vi "Robot Global Data.vi"() -> ()   [LabVIEW 2017]
doc: "This global VI can contain as many global variables as you need. Place a control on the panel, give it a good name. To read or write to it from a VI, drag the icon to the diagram of that VI. You can also drag from the project. Click on the node to change which global you access. You shouldn't have multiple locations writing to a global or it will cause a race-condition."
uses:
  <vilib>/Rock Robotics/WPI/Camera/WPI_CameraImageSize.ctl
  <vilib>/Rock Robotics/WPI/DriverStation/WPI_DriverStationRobotMode2.ctl
panel:
  in  "SweetSpot":dbl=0.4
  out "WristSet":dbl
  out "LiftSet":dbl
  out "TempWrist":dbl
  out "WristVelocity":dbl
  out "WristDistance":dbl
  in  "WristDistanceArr":dbl[](array[numeric])
  in  "WristVelocityArr":dbl[](array[numeric])
  out "LiftVelocity":dbl
  out "LiftDistance":dbl
  in  "LiftDistanceArr":dbl[](array[numeric])
  in  "LiftVelocityArr":dbl[](array[numeric])
  in  "Cube Found?":bool
  in  "LiftSet?":bool
  out "AvgVel":dbl
  out "AvgDist":dbl
  out "YawVelocity":dbl
  out "Yaw":dbl
  in  "NavXArr":dbl[](array[numeric])
  out "RightVelocity":dbl
  out "RightDistance":dbl
  out "LeftVelocity":dbl
  out "LeftDistance":dbl
  in  "RightDistanceArr":dbl[](array[numeric])
  in  "LeftDistanceArr":dbl[](array[numeric])
  in  "RightVelocityArr":dbl[](array[numeric])
  in  "LeftVelocityArr":dbl[](array[numeric])
  out "IntakeTime":dbl
  out "IntakeSwitch":dbl
  out "IntakeCount":dbl
  out "OppSwitch":dbl
  out "Scale":dbl
  out "Switch":dbl
  out "Limelight":cluster{"tx":dbl, "ty":dbl, "ta":dbl, "ts":dbl}
  out "Optical True":bool
  in  "Robot Mode":T1
  in  "image size":T2=enum."320x240"
  in  "Enable Vision":bool
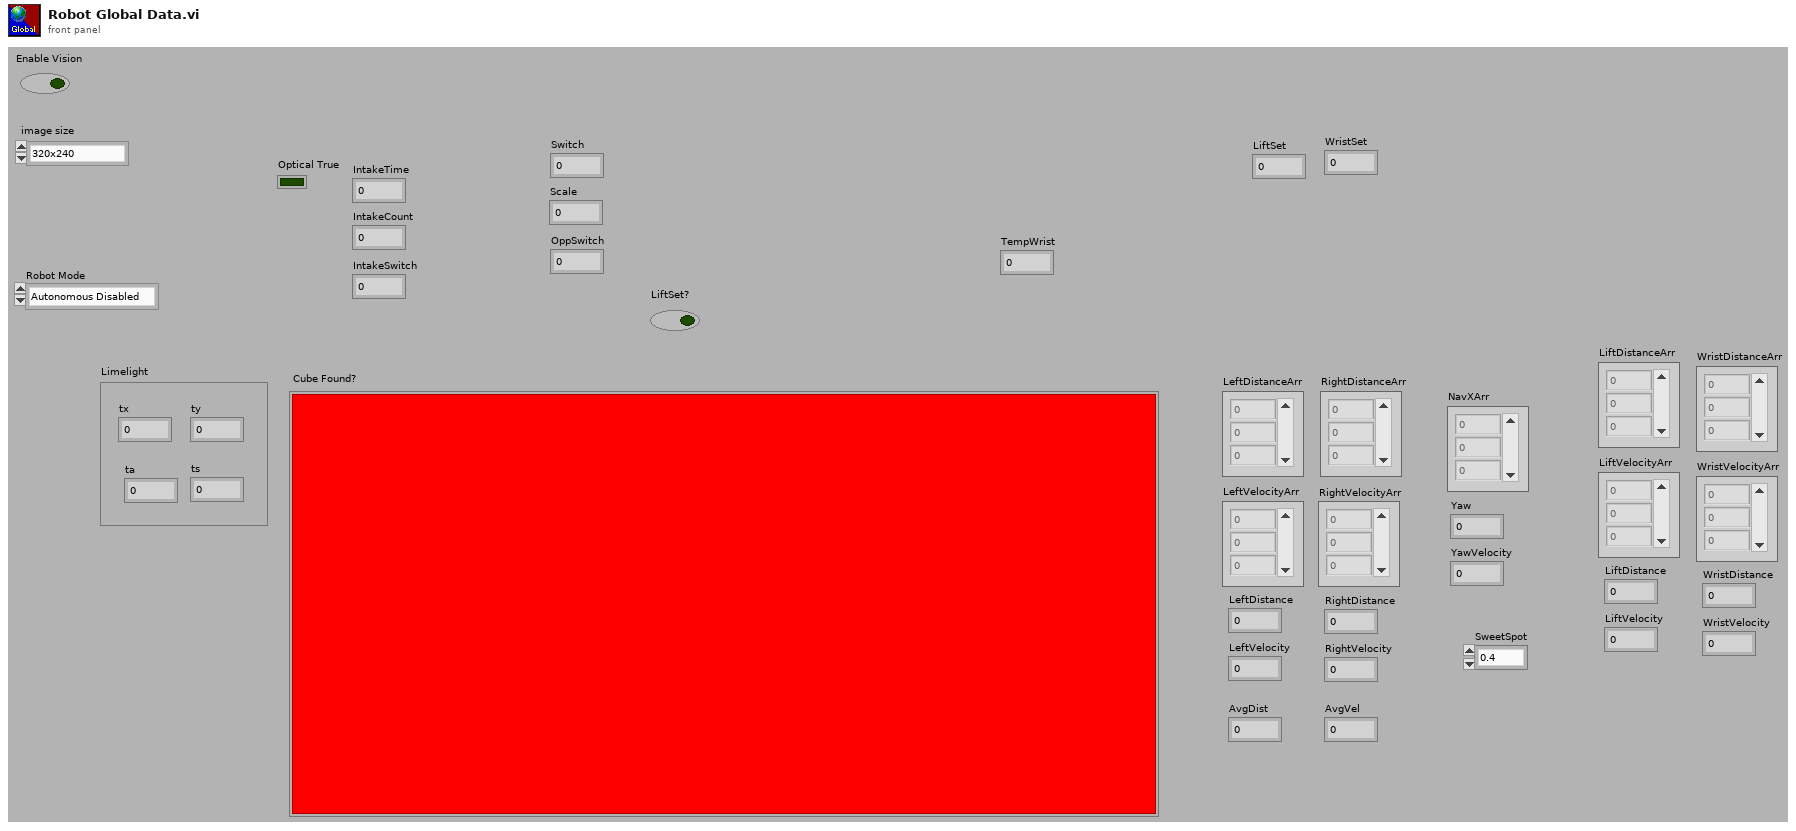
[diagram p1: front panel]
types:
  T1 = typedef "WPI_DriverStationRobotMode2.ctl" = enum16{"Autonomous Disabled", "Autonomous Enabled", "Teleop Disabled", "Teleop Enabled", "Disconnected", "Finish", "Test Disabled", "Test Enabled", "Emergency Stopped"}
  T2 = typedef "WPI_CameraImageSize.ctl" = enum16{"640x480", "320x240", "160x120", "Custom"}
diagram:
